vi "ExpLogInit.vi"   [LabVIEW 2019]
types:
  T1 = enum16{"open", "replace", "create", "open or create", "replace or create", "replace or create with confirmation"}
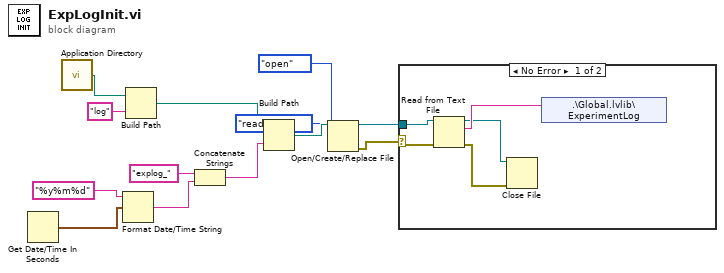
[diagram p0: block diagram]
diagram:
  n1 = Get Date/Time In Seconds() -> (seconds since 1Jan1904=w12:timestamp)
  n2 = call <vilib>:"Application Directory.vi"() -> ("Application Directory"=w11:path)
  n3 = Format Date/Time String(time format string (%c)="%y%m%d", seconds (now)=w12) -> (date/time string=w9:string)  [unwired: 1 in]
  n4 = Build Path(base path=w11, name or relative path="log") -> (appended path=w7:path)
  n5 = Concatenate Strings("explog_" ("string"), w9) -> (w6:string)
  n6 = Build Path(base path=w7, name or relative path=w6) -> (appended path=w5:path)
  n7 = Open/Create/Replace File(file path (use dialog)=w5, operation (0:open)=T1."open", access (0:read/write)=enum16{"read/write", "read-only", "write-only"}."read-only") -> (refnum out=w1:refnum<file>, error out=w3:errorcluster)  [unwired: 3 in, 1 out]
  n8 = case shown="No Error" w3 {
    selector: w3 -> [w17 _]
    tunnel: w1 -> [w18 _]
    frame No Error {
      n9 = Read from Text File(file (use dialog)=w18, error in=w17) -> (refnum out=w15:refnum<file>, text=w16:string, error out=w14:errorcluster)  [unwired: 2 in, 1 out]
      n10 = Close File(refnum=w15, error in=w14) -> ()  [unwired: 2 out]
      n11 = shared-variable ".\\Global.lvlib\\ExperimentLog"(w16) -> ()  [unwired: 1 in, 1 out]
    }
    frame Error {
    }
  }
